vi "Normalized Axes.vi"(8 "axis info in":T2, 11 "axis info":T3) -> (0 "axis info out":T1)   [LabVIEW 2012]
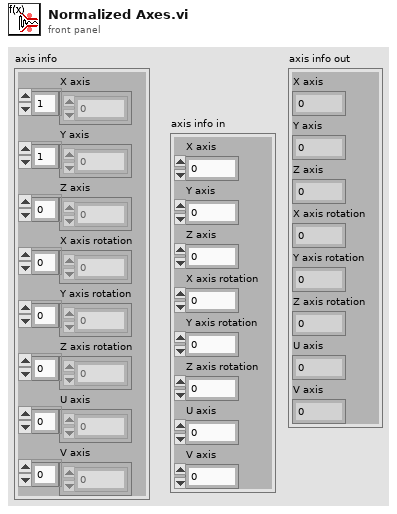
[diagram p1: front panel]
types:
  T1 = cluster{"X axis":dbl, "Y axis":dbl, "Z axis":dbl, "X axis rotation":dbl, "Y axis rotation":dbl, "Z axis rotation":dbl, "U axis":dbl, "V axis":dbl}
  T2 = cluster{"X axis":i32, "Y axis":i32, "Z axis":i32, "X axis rotation":i32, "Y axis rotation":i32, "Z axis rotation":i32, "U axis":i32, "V axis":i32}
  T3 = cluster{"X axis":dbl[], "Y axis":dbl[], "Z axis":dbl[], "X axis rotation":dbl[], "Y axis rotation":dbl[], "Z axis rotation":dbl[], "U axis":dbl[], "V axis":dbl[]}
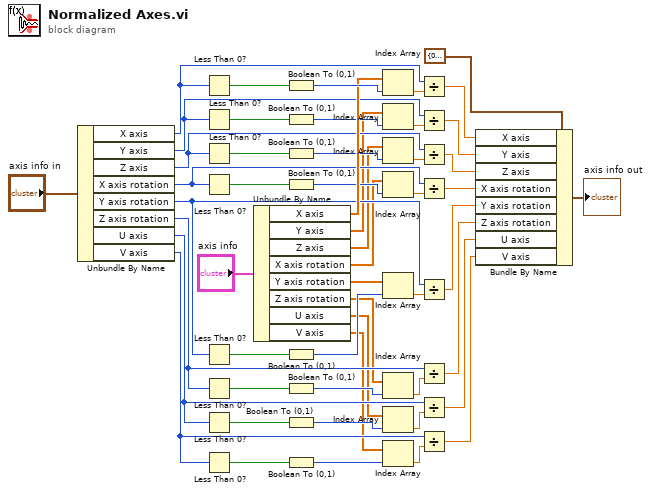
[diagram p0: block diagram]
diagram:
  n1 = Unbundle By Name("axis info in") -> ("X axis"=w46:i32, "Y axis"=w14:i32, "Z axis"=w13:i32, "X axis rotation"=w12:i32, "Y axis rotation"=w11:i32, "Z axis rotation"=w10:i32, "U axis"=w9:i32, "V axis"=w8:i32)
  n2 = Less Than 0?(x=w46) -> (x < 0?=w50:bool)
  n3 = Less Than 0?(x=w14) -> (x < 0?=w40:bool)
  n4 = Less Than 0?(x=w13) -> (x < 0?=w39:bool)
  n5 = Less Than 0?(x=w12) -> (x < 0?=w34:bool)
  n6 = Less Than 0?(x=w11) -> (x < 0?=w33:bool)
  n7 = Less Than 0?(x=w10) -> (x < 0?=w28:bool)
  n8 = Less Than 0?(x=w9) -> (x < 0?=w27:bool)
  n9 = Less Than 0?(x=w8) -> (x < 0?=w16:bool)
  n10 = Unbundle By Name("axis info") -> ("X axis"=w48:dbl[], "Y axis"=w7:dbl[], "Z axis"=w6:dbl[], "X axis rotation"=w5:dbl[], "Y axis rotation"=w4:dbl[], "Z axis rotation"=w3:dbl[], "U axis"=w2:dbl[], "V axis"=w1:dbl[])
  n11 = Boolean To (0,1)(Boolean=w50) -> (0, 1=w49:i16)
  n12 = Boolean To (0,1)(Boolean=w40) -> (0, 1=w41:i16)
  n13 = Boolean To (0,1)(Boolean=w39) -> (0, 1=w38:i16)
  n14 = Boolean To (0,1)(Boolean=w34) -> (0, 1=w35:i16)
  n15 = Boolean To (0,1)(Boolean=w33) -> (0, 1=w32:i16)
  n16 = Boolean To (0,1)(Boolean=w28) -> (0, 1=w29:i16)
  n17 = Boolean To (0,1)(Boolean=w27) -> (0, 1=w26:i16)
  n18 = Boolean To (0,1)(Boolean=w16) -> (0, 1=w17:i16)
  n19 = Index Array(array=w48, index=w49) -> (element=w47:dbl)
  n20 = Index Array(array=w7, index=w41) -> (element=w42:dbl)
  n21 = Index Array(array=w6, index=w38) -> (element=w37:dbl)
  n22 = Index Array(array=w5, index=w35) -> (element=w36:dbl)
  n23 = Index Array(array=w4, index=w32) -> (element=w31:dbl)
  n24 = Index Array(array=w3, index=w29) -> (element=w30:dbl)
  n25 = Index Array(array=w2, index=w26) -> (element=w25:dbl)
  n26 = Index Array(array=w1, index=w17) -> (element=w18:dbl)
  n27 = Divide(x=w46, y=w47) -> (x/y=w43:dbl)
  n28 = Divide(x=w14, y=w42) -> (x/y=w24:dbl)
  n29 = Divide(x=w13, y=w37) -> (x/y=w23:dbl)
  n30 = Divide(x=w12, y=w36) -> (x/y=w22:dbl)
  n31 = Divide(x=w11, y=w31) -> (x/y=w21:dbl)
  n32 = Divide(x=w10, y=w30) -> (x/y=w20:dbl)
  n33 = Divide(x=w9, y=w25) -> (x/y=w19:dbl)
  n34 = Divide(x=w8, y=w18) -> (x/y=w15:dbl)
  n35 = Bundle By Name(cluster=T1 {"X axis"=0.0, "Y axis"=0.0, "Z axis"=0.0, "X axis rotation"=0.0, "Y axis rotation"=0.0, "Z axis rotation"=0.0, "U axis"=0.0, "V axis"=0.0} ("axis info out"), "X axis"=w43, "Y axis"=w24, "Z axis"=w23, "X axis rotation"=w22, "Y axis rotation"=w21, "Z axis rotation"=w20, "U axis"=w19, "V axis"=w15) -> (→"axis info out":T1)
